vi "Main.vi"() -> ()   [LabVIEW 2026]
doc: "This Continuous Measurement sample project is based on the Queued Message Handler template.\n\nThe Event Handling Loop generates messages based on user interface actions.\n\nThe Message Handling Loop processes messages generated by the Event Handling Loop, or by other messages. There are also Acquisition and Logging message handling loop subVIs, and a chart updating loop."
uses:
  controls/Messaging Payloads/Sensor CoreData.ctl
  controls/Messaging Payloads/Sensor CoreData Cluster.ctl
  controls/UI/Units Enum.ctl
  controls/UI/Signal Enum.ctl
  controls/UI/Settings Cluster.ctl
  controls/UI/Acq Settings.ctl
  Acquisition/Instrument Specifications Configuration.ctl
  Acquisition/Instrument Specifications Cluster Configuration.ctl
  controls/UI/Measurement Role.ctl
  controls/UI/Config Settings.ctl
  Processing/Processing Settings.ctl
  Processing/Test Parameters.ctl
  Processing/Test Parameters Cluster.ctl
  controls/UI/Test Sequence Context.ctl
  controls/UI/Test Sequence Context Cluster.ctl
  controls/UI/Direction.ctl
  controls/UI/Session Identfiers.ctl
  controls/UI/Test Sequence Settings.ctl
  controls/UI/Test Sequence State.ctl
  controls/UI/Test Sequence Enum.ctl
  controls/Controller/Stimulus Settings.ctl
  controls/Controller/Stimulus Outputs.ctl
  controls/Controller/Stimulus Output.ctl
  controls/Controller/Controller Core Data.ctl
  controls/Controller/Stimulus Output Configuration.ctl
  controls/Controller/Stimulus Role.ctl
  controls/UI/UI Data.ctl
  controls/UI/UI State.ctl
  controls/UI/System Config.ctl
  controls/UI/Analog Output.ctl
  Acquisition/Acquisition Payload.ctl
  Acquisition/Acquisition Context.ctl
  support/Architecture/Message Queue/Enqueue Message (Single).vi
  support/Architecture/Message Queue/Enqueue Message (Array).vi
  <vilib>/Utility/error.llb/Error Cluster From Error Code.vi
  <vilib>/ErrorRing/Error Ring.xnode
  support/Architecture/User Event - Stop/User Event - Stop.lvlib
  support/Architecture/Message Queue/Message Queue.lvlib
  Settings/Settings Dialog.vi
  Settings/Settings.lvlib
  Database/Database.lvlib
  Logging/Logging.lvlib
  Processing/Processing_Engine.lvlib
  Acquisition/Acquisition.lvlib
  support/UI Utilities/Login.vi
  Analysis/Analysis Dialog.vi
  Analysis/Analysis.lvlib
panel:
  in  "Stop":bool
  in  "Start":bool
  out "Sensor Information":T1
  in  "Generate Analytics":bool
  in  "Simulation Mode":bool
  in  "Manage Serial Numbers":bool
  out "Data":waveform(dbl)[](graph)
  in  "Settings":bool
  out "Status":string
  in  "Exit":bool
  # "OFF"
  # "Automated Safety Calibration Rig"
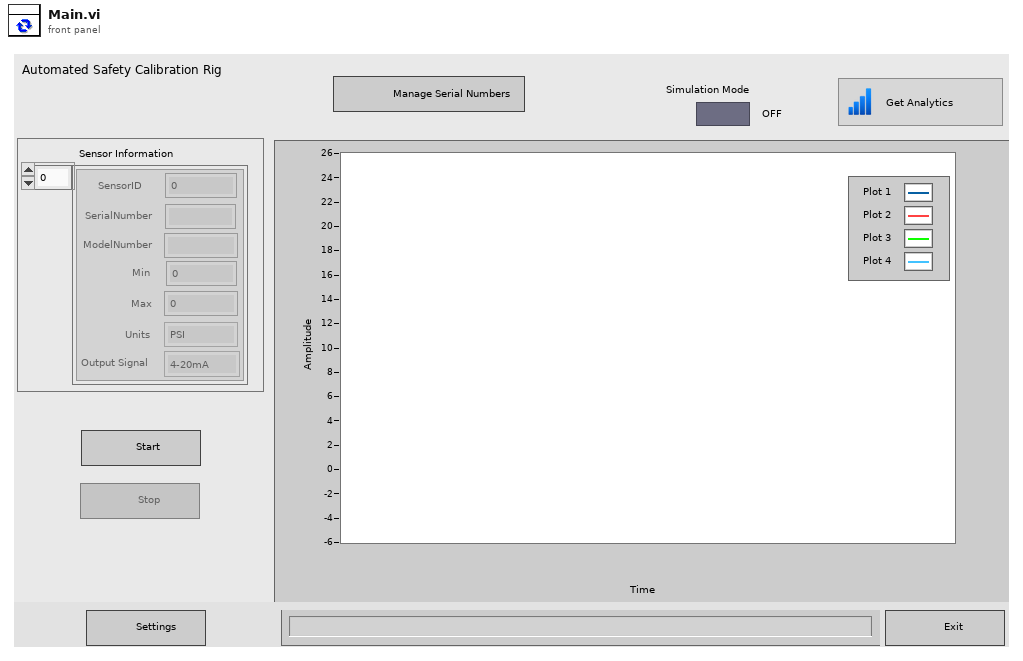
[diagram p1: front panel]
types:
  T1 = typedef "Sensor CoreData.ctl" = T2[]
  T2 = typedef "Settings.lvlib/Sensor CoreData Cluster.ctl" = cluster{"SensorID":i32, "SerialNumber":string, "ModelNumber":string, "Min":dbl, "Max":dbl, "Units":T3, "Output Signal":T4}
  T3 = typedef "Units Enum.ctl" = enum16{"PSI", "Deg C", "kPa", "GPM"}
  T4 = typedef "Signal Enum.ctl" = enum16{"4-20mA", "0-10V", "Thermocouple Type K"}
  T5 = typedef "System Config.ctl" = cluster{"AdminHash":string, "LogFileBasePath ":path, "Config Settings":T6, "AnalogOutput":T7}
  T6 = typedef "Config Settings.ctl" = cluster{"Simulated Sensor Injection":dbl, "Base Device Name":string, "Simulation Mode":string}
  T7 = typedef "Settings.lvlib/Analog Output.ctl" = cluster{"Pressure Controller":string, "Temperature Controller":string}
  T8 = typedef "UI State.ctl" = enum16{"Idle", "Acquiring and Logging", "Waiting for Exit", "Waiting for Exit (Acq Stopped)", "Waiting for Exit (Log Stopped)", "Waiting for Stop", "Waiting for Stop (Acq Stopped)", "Waiting for Stop (Log Stopped)"}
  T9 = typedef "UI Data.ctl" = cluster{"Start Ref":refnum<vi>, "Stop Ref":refnum<vi>, "Settings Ref":refnum<vi>, "Exit Ref":refnum<vi>, "Status Ref":refnum<vi>, "Data Ref":refnum<vi>, "Sim  Refnum":refnum<vi>}
  T10 = typedef "Settings Cluster.ctl" = cluster{"Acq Settings":T11, "Processing Settings":T15, "Session Identifiers":T21, "Test Sequence Settings":T22, "Stimulus Settings":T25}
  T11 = typedef "Acq Settings.ctl" = cluster{"Instrument Specifications":T12, "Config Settings":T6}
  T12 = typedef "Acquisition.lvlib/Instrument Specifications Configuration.ctl" = T13[]
  T13 = typedef "Acquisition.lvlib/Instrument Specifications Cluster Configuration.ctl" = cluster{"Sensor ID":i32, "Target Sample Rate (Hz)":dbl, "Steady-State Duration (s)":i32, "Allowed Tolerance (%) FS":dbl, "Max Settling Timeout (s)":i32, "Physical Channel":string, "Measurement Role":T14}
  T14 = typedef "Settings.lvlib/Measurement Role.ctl" = enum16{"Controller", "Reference", "UUT", "Disable", "All"}
  T15 = typedef "Processing_Engine.lvlib/Processing Settings.ctl" = cluster{"Sensor CoreData":T1, "Test Parameters":T16, "Measurement Roles":T14[], "Test Sequence Context":T18}
  T16 = typedef "Processing_Engine.lvlib/Test Parameters.ctl" = T17[]
  T17 = typedef "Settings.lvlib/Test Parameters Cluster.ctl" = cluster{"Steady-State Duration (s)":i32, "Allowed Tolerance (%) FS":dbl, "Max Settling Timeout (s)":i32}
  T18 = typedef "Settings.lvlib/Test Sequence Context.ctl" = T19[]
  T19 = typedef "Settings.lvlib/Test Sequence Context Cluster.ctl" = cluster{"Direction":T20, "Cycle Number":i32}
  T20 = typedef "Settings.lvlib/Direction.ctl" = enum16{"Acsending", "Descending"}
  T21 = typedef "Session Identfiers.ctl" = cluster{"SerialNumber":string[], "OperatorName":string}
  T22 = typedef "Test Sequence Settings.ctl" = cluster{"Test Sequence State":T23}
  T23 = typedef "Settings.lvlib/Test Sequence State.ctl" = cluster{"Test Sequence Enum":T24, "Point Index":i32, "Current Target":dbl, "Previous Target":dbl, "Simulation?":bool, "Direction":T20, "Transition Active?":bool, "Cycle Number":i32}
  T24 = typedef "Test Sequence Enum.ctl" = enum16{"Idle", "Start Point", "Point Complete", "Test Complete", "Abort Test", "Reset"}
  T25 = typedef "Settings.lvlib/Stimulus Settings.ctl" = cluster{"Stimulus Outputs":T26}
  T26 = typedef "Settings.lvlib/Stimulus Outputs.ctl" = T27[]
  T27 = typedef "Settings.lvlib/Stimulus Output.ctl" = cluster{"Controller Core Data":T28, "Stimulus Output Configuration":T29}
  T28 = typedef "Settings.lvlib/Controller Core Data.ctl" = cluster{"Min":dbl, "Max":dbl, "Units":T3, "Input Signal Type":T4, "Input Signal Min":dbl, "Input Signal Max":dbl}
  T29 = typedef "Settings.lvlib/Stimulus Output Configuration.ctl" = cluster{"DAQmx AO Physical Channel":tag, "Role":T30, "Model Numbers":string, "Serial Numbers":string}
  T30 = typedef "Stimulus Role.ctl" = enum16{"Pressure Controller", "Temperature Controller"}
  T31 = typedef "Message Queue.lvlib/All Message Queues.ctl" = cluster{"UI":refnum<queue>, "Database":refnum<queue>, "Processing":refnum<queue>, "Acquisition":refnum<queue>, "Logging":refnum<queue>, "Analysis":refnum<queue>}
  T32 = enum8{"Enabled", "Disabled", "Disabled and Grayed Out"}
  T33 = typedef "Acquisition.lvlib/Acquisition Payload.ctl" = cluster{"Acq Settings":T11, "Acquisition Context":T34, "Stimulus Settings":T25}
  T34 = typedef "Acquisition.lvlib/Acquisition Context.ctl" = cluster{"Setpoint":dbl, "Previous Setpoint":dbl, "Transition Start Time":dbl, "Transition Active?":bool}
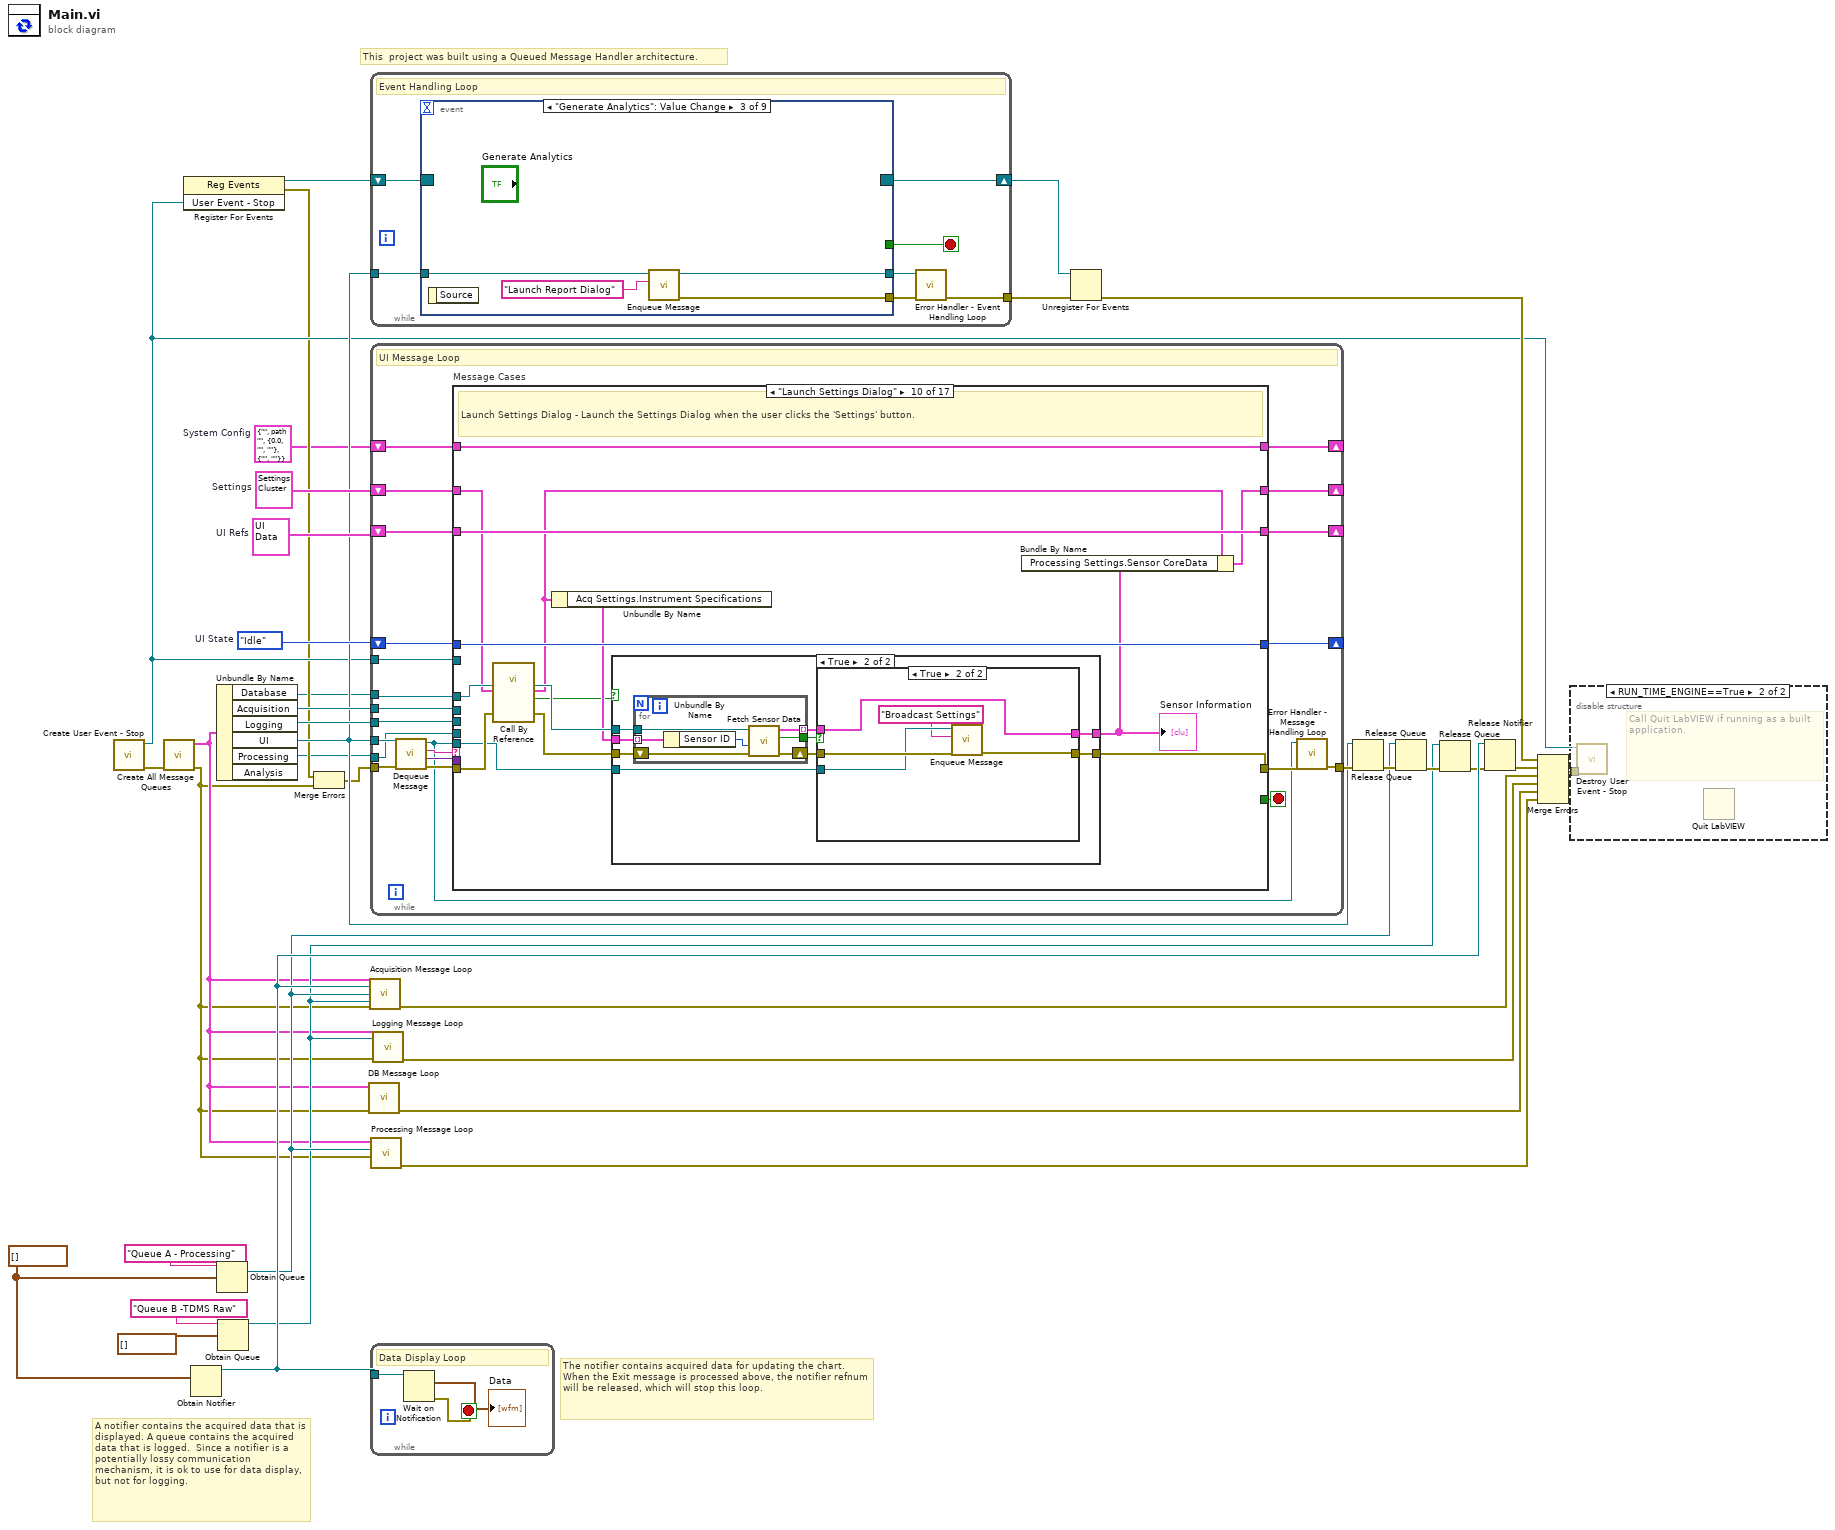
[diagram p0: block diagram]
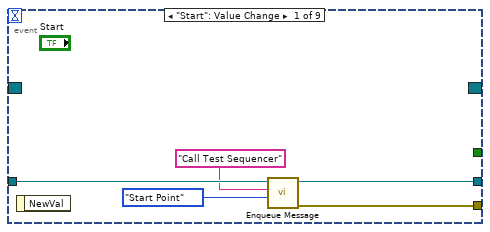
[diagram p3: hidden frame]
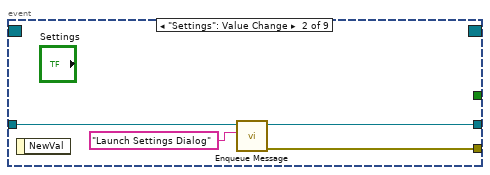
[diagram p4: hidden frame]
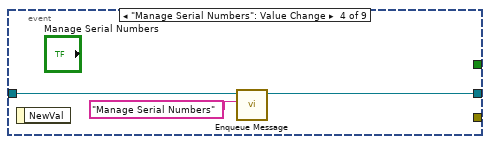
[diagram p5: hidden frame]
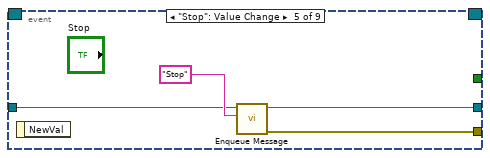
[diagram p6: hidden frame]
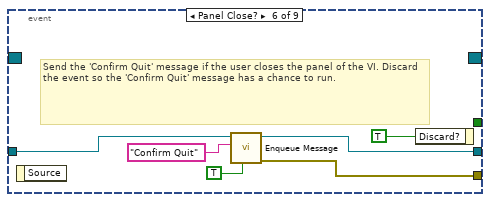
[diagram p7: hidden frame]
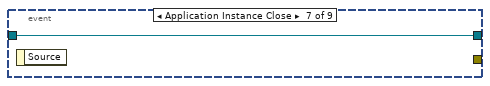
[diagram p8: hidden frame]
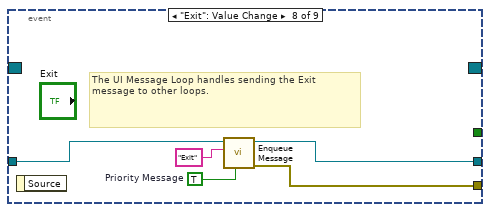
[diagram p9: hidden frame]
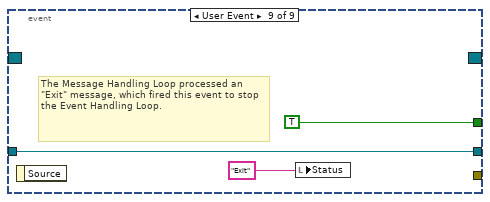
[diagram p10: hidden frame]
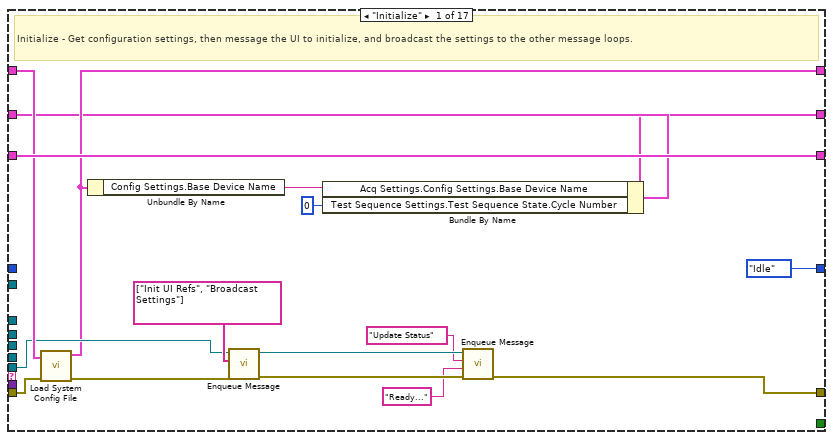
[diagram p11: hidden frame]
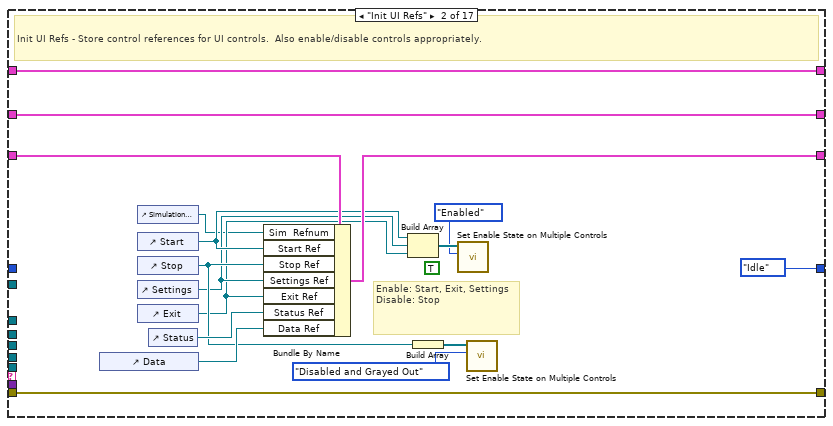
[diagram p12: hidden frame]
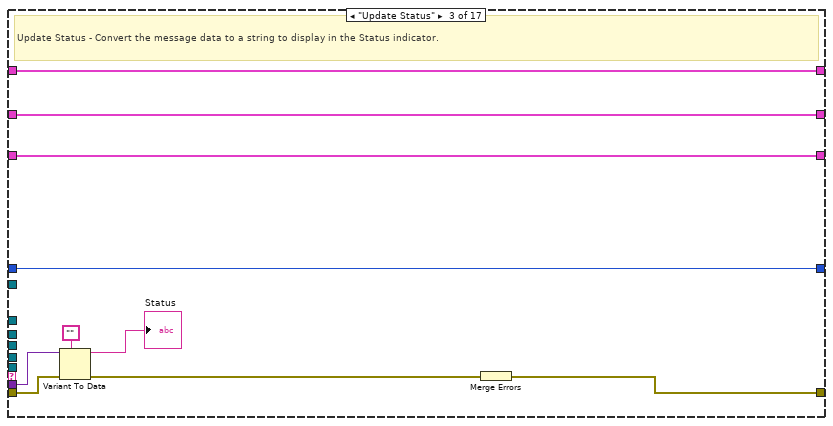
[diagram p13: hidden frame]
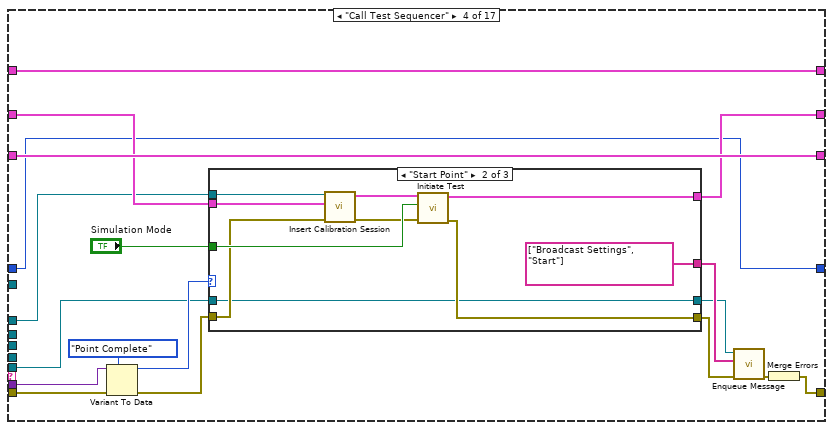
[diagram p14: hidden frame]
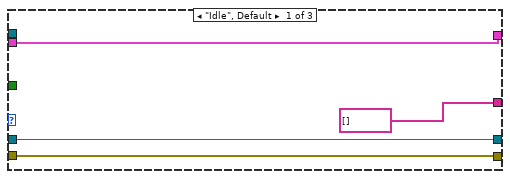
[diagram p15: hidden frame]
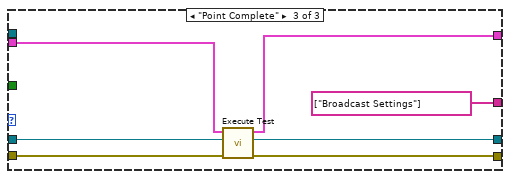
[diagram p16: hidden frame]
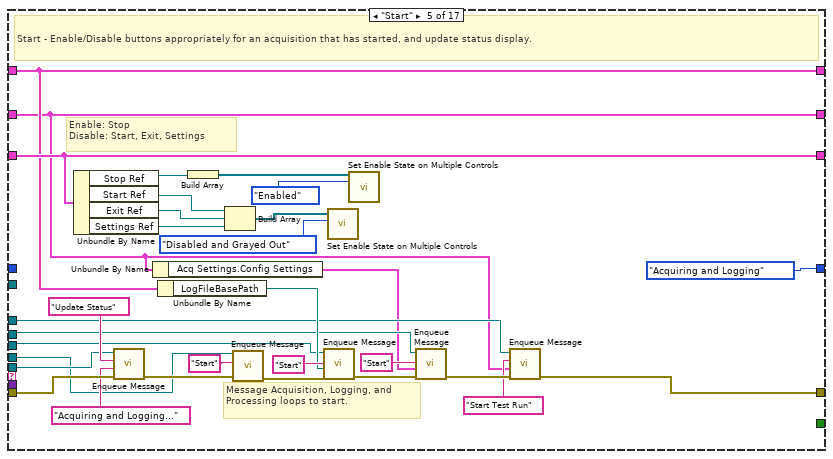
[diagram p17: hidden frame]
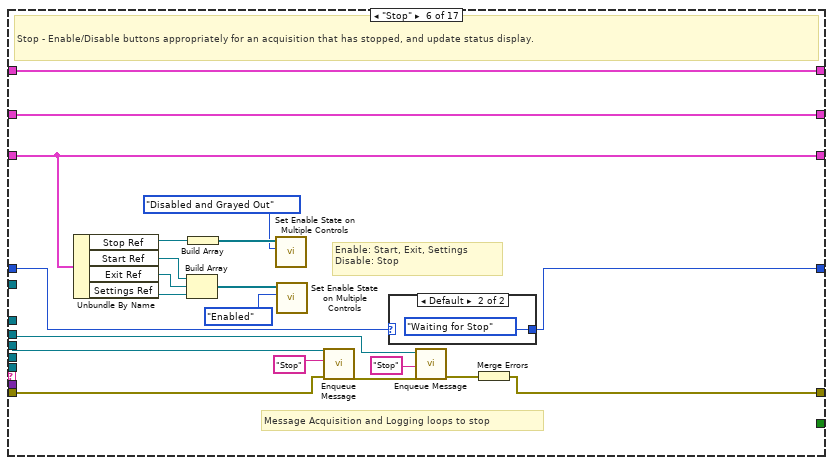
[diagram p18: hidden frame]
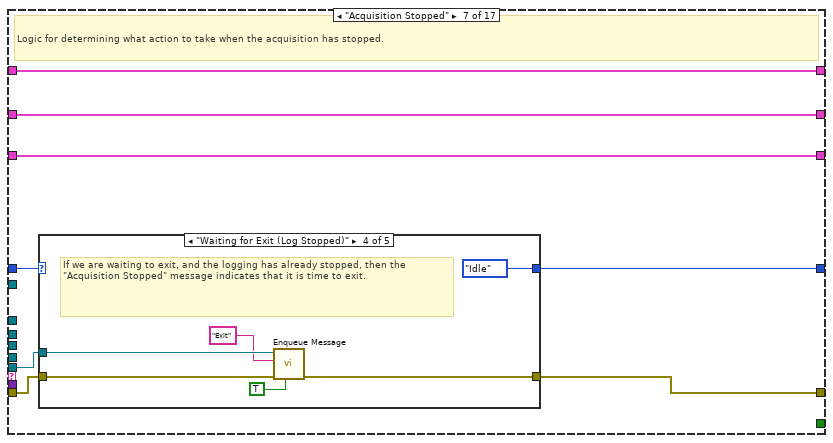
[diagram p20: hidden frame]
diagram:
  w14 = T5 {"AdminHash"="", "LogFileBasePath "=path "", "Config Settings"={"Simulated Sensor Injection"=0.0, "Base Device Name"="", "Simulation Mode"=""}, "AnalogOutput"={"Pressure Controller"="", "Temperature Controller"=""}}  # System Config
  w26 = UI_State."Idle"  # UI State
  w6 = waveform(dbl)[] []
  w29 = T9 {"Start Ref"=refnum, "Stop Ref"=refnum, "Settings Ref"=refnum, "Exit Ref"=refnum, "Status Ref"=refnum, "Data Ref"=refnum, "Sim  Refnum"=refnum}  # UI Refs
  w32 = T10 {"Acq Settings"={"Instrument Specifications"=[], "Config Settings"={"Simulated Sensor Injection"=0.0, "Base Device Name"="", "Simulation Mode"=""}}, "Processing Settings"={"Sensor CoreData"=[], "Test Parameters"=[], "Measurement Roles"=[], "Test Sequence Context"=[]}, "Session Identifiers"={"SerialNumber"=[], "OperatorName"=""}, "Test Sequence Settings"={"Test Sequence State"={"Test Sequence Enum"=enum."Idle", "Point Index"=0, "Current Target"=0.0, "Previous Target"=0.0, "Simulation?"=FALSE, "Direction"=enum."Acsending", "Transition Active?"=FALSE, "Cycle Number"=0}}, "Stimulus Settings"={"Stimulus Outputs"=[]}}  # Settings
  # "This  project was built using a Queued Message Handler architecture."
  # "A notifier contains the acquired data that is displayed. A queue contains the acquired data that is logged.  Since a notifier is a potentially lossy communication mechanism, it is ok to use for data display, but not for logging."
  # "The notifier contains acquired data for updating the chart. When the Exit message is processed above, the notifier refnum will be released, which will stop this loop."
  n1 = call "Create User Event - Stop.vi"() -> ("error out"=w34:errorcluster, "User Event - Stop"=w19:refnum<user-event>)  [unwired: 10 in]
  n2 = call "Create All Message Queues.vi"("error in (no error)"=w34) -> ("error out"=w1:errorcluster, "Message Queues out"=w2:T31)  [unwired: 9 in]
  n3 = register-events(w19) -> (reference out=w20:refnum<event-registration>, error out=w17:errorcluster)  [unwired: 2 in]
  n4 = Obtain Notifier(notification data type=w6) -> (notifier out=w8:refnum<notifier>)  [unwired: 3 in, 2 out]
  n5 = Unbundle By Name(w2) -> ("Database"=w15:refnum<queue>, "Acquisition"=w28:refnum<queue>, "Logging"=w27:refnum<queue>, "UI"=w24:refnum<queue>, "Processing"=w13:refnum<queue>)  [unwired: 1 out]
  n6 = Obtain Queue(name (unnamed)="Queue A - Processing", element data type=w6) -> (queue out=w7:refnum<queue>)  [unwired: 3 in, 2 out]
  n7 = Obtain Queue(name (unnamed)="Queue B -TDMS Raw", element data type=waveform(dbl)[] []) -> (queue out=w3:refnum<queue>)  [unwired: 3 in, 2 out]
  n8 = Merge Errors(w17, w1) -> (w18:errorcluster)
  n9 = call "DB Message Loop.vi"("error in (no error)"=w1, "Message Queues"=w2) -> ("error out"=w16:errorcluster)  [unwired: 9 in]
  n10 = call "Acquisition Message Loop.vi"("Message Queues"=w2, "Data Notifier"=w8, "Queue A - Processing"=w7, "Queue B -TDMS Raw"=w3, "error in (no error)"=w1) -> ("error out"=w35:errorcluster)  [unwired: 10 in]
  n11 = while {
    tunnel: w24 -> [w43]
    tunnel: [w40] -> w36
    shift-right: [w42] -> w30
    shift-left: w20 -> [w44]
    stop <- w41 stop-if-true
    # "Event Handling Loop"
    n12 = event shown="[2] \"Generate Analytics\": Value Change" {
      selector: w44 -> [_ _ _ _ _ _ _ _ _]
      dyn-events: [_ _ _ _ _ _ _ _ _] -> w42
      timeout: _ -> [_ _ _ _ _ _ _ _ _]
      tunnel: [_ _ _ _ _ _ _ _ TRUE ("Discard?")] -> w41
      tunnel: w43 -> [w49 w52 w56 w59 w63 w68 w71 w73 w77]
      tunnel: [w47 w50 w54 _ w62 w66 _ w76 _] -> w39
      tunnel: [w46 w51 w55 w58 w61 w67 w71 w72 w77] -> w38
      event "Start": Value Change {
        n13 = event-data() -> ()  [unwired: 1 in, 1 out]
        n14 = call-poly "Enqueue Message.vi"("Message Data"=Test_Sequence_Enum."Start Point" ("Test Sequence State.Test Sequence Enum"), "Message"="Call Test Sequencer", "Message Queue"=w49) -> ("error out"=w47:errorcluster, "dup Message Queue"=w46:refnum<queue>)  [unwired: 7 in]
      }
      event "Settings": Value Change {
        n15 = event-data() -> ()  [unwired: 1 in, 1 out]
        n16 = call-poly "Enqueue Message.vi"("Message"="Launch Settings Dialog", "Message Queue"=w52) -> ("error out"=w50:errorcluster, "dup Message Queue"=w51:refnum<queue>)  [unwired: 8 in]
      }
      event "Generate Analytics": Value Change {
        n17 = event-data() -> ()  [unwired: 1 in, 1 out]
        n18 = call-poly "Enqueue Message.vi"("Message"="Launch Report Dialog", "Message Queue"=w56) -> ("error out"=w54:errorcluster, "dup Message Queue"=w55:refnum<queue>)  [unwired: 8 in]
      }
      event "Manage Serial Numbers": Value Change {
        n19 = event-data() -> ()  [unwired: 1 in, 1 out]
        n20 = call-poly "Enqueue Message.vi"("Message"="Manage Serial Numbers", "Message Queue"=w59) -> ("dup Message Queue"=w58:refnum<queue>)  [unwired: 8 in, 1 out]
      }
      event "Stop": Value Change {
        n21 = event-data() -> ()  [unwired: 1 in, 1 out]
        n22 = call-poly "Enqueue Message.vi"("Message"="Stop", "Message Queue"=w63) -> ("error out"=w62:errorcluster, "dup Message Queue"=w61:refnum<queue>)  [unwired: 8 in]
      }
      event Panel Close? {
        # "Send the 'Confirm Quit' message if the user closes the panel of the VI. Discard the event so the 'Confirm Quit' message has a chance to run."
        n23 = event-data() -> ()  [unwired: 1 in, 1 out]
        n24 = call-poly "Enqueue Message.vi"("Priority Message? (F)"=TRUE, "Message"="Confirm Quit", "Message Queue"=w68) -> ("error out"=w66:errorcluster, "dup Message Queue"=w67:refnum<queue>)  [unwired: 7 in]
        n25 = event-data("Discard?"=TRUE) -> ()  [unwired: 1 in, 1 out]
      }
      event Application Instance Close {
        n26 = event-data() -> ()  [unwired: 1 in, 1 out]
      }
      event "Exit": Value Change {
        w74 = TRUE  # Priority Message
        # "The UI Message Loop handles sending the Exit message to other loops."
        n27 = event-data() -> ()  [unwired: 1 in, 1 out]
        n28 = call-poly "Enqueue Message.vi"("Priority Message? (F)"=w74, "Message"="Exit", "Message Queue"=w73) -> ("error out"=w76:errorcluster, "dup Message Queue"=w72:refnum<queue>)  [unwired: 7 in]
      }
      event User Event {
        # "The Message Handling Loop processed an \"Exit\" message, which fired this event to stop the Event Handling Loop."
        n29 = event-data() -> ()  [unwired: 1 in, 1 out]
        n30 = local write "Status"("Exit" ("Exit String")) -> ()
      }
    }
    n31 = call "Error Handler - Event Handling Loop.vi"("error in (no error)"=w39, "Message Queue"=w38) -> ("dup error in"=w40:errorcluster)  [unwired: 8 in, 1 out]
  }
  n32 = while {
    tunnel: w24 -> [w95]
    tunnel: w19 -> [w100]
    shift-right: [w94] -> _
    shift-left: w32 -> [w93]
    shift-right: [w91] -> _
    shift-left: w29 -> [w92]
    tunnel: w28 -> [w90]
    tunnel: w27 -> [w89]
    shift-right: [w84] -> _
    shift-left: w26 -> [w85]
    tunnel: w18 -> [w99]
    tunnel: [w88] -> w37
    tunnel: w15 -> [w83]
    shift-right: [w81] -> _
    shift-left: w14 -> [w82]
    tunnel: w13 -> [w80]
    stop <- w101 stop-if-true
    # "UI Message Loop"
    n33 = call "Dequeue Message.vi"("error in (no error)"=w99, "Message Queue"=w95) -> ("error out"=w98:errorcluster, "Message Data"=w96:variant, "Message"=w97:string, "dup Message Queue"=w86:refnum<queue>)  [unwired: 6 in]
    n34 = case "Message Cases" shown="\"Launch Settings Dialog\"" w97 {
      selector: w97 -> [_ _ _ _ _ _ _ _ _ _ _ _ _ _ _ _ w438]
      tunnel: w86 -> [w109 _ _ w148 w192 _ w242 w268 _ w313 _ w368 _ w384 _ _ _]
      tunnel: w98 -> [w111 w135 w144 w163 w215 w236 w243 w269 w302 w326 w359 w369 w371 w383 w415 w435 _]
      tunnel: [w103 w135 w145 w157 w195 w216 w240 w266 w311 w322 w355 w364 w374 w382 w427 w434 w437] -> w87
      tunnel: [_ _ _ _ _ _ _ _ _ _ _ _ _ _ TRUE _ _] -> w101
      tunnel: w96 -> [_ _ w143 w162 _ _ _ _ _ _ _ _ w375 _ w420 _ _]
      tunnel: w100 -> [_ _ _ _ _ _ _ _ _ _ _ _ _ _ w428 _ _]
      tunnel: [w104 w134 w139 w158 w186 w235 w246 w272 w292 w314 w354 w361 w379 w387 w426 w433 w441] -> w94
      tunnel: w93 -> [w105 w134 w139 w156 w186 w235 w246 w272 w301 w320 w354 w361 w379 w387 w426 w433 w441]
      tunnel: w92 -> [w114 w133 w138 w161 w213 w234 w245 w271 w310 w324 w358 w366 w378 w386 w425 w432 w440]
      tunnel: [w114 w130 w138 w161 w213 w234 w245 w271 w310 w324 w358 w366 w378 w386 w425 w432 w440] -> w91
      tunnel: w90 -> [_ _ _ _ w191 w223 _ _ w300 _ _ _ _ _ w417 _ _]
      tunnel: w89 -> [_ _ _ _ w190 w226 _ _ _ _ _ _ _ _ w424 _ _]
      tunnel: w85 -> [_ _ w137 w155 _ w220 w244 w270 w309 w323 w357 w365 w373 w385 _ w431 w439]
      tunnel: [UI_State."Idle" ("UI State") UI_State."Idle" ("UI State") w137 w155 UI_State."Acquiring and Logging" ("UI State") w221 w241 w267 w309 w323 w357 w365 w373 w381 UI_State."Idle" ("UI State") w431 w439] -> w84
      tunnel: w83 -> [_ _ _ w146 w193 _ _ _ _ w321 w353 w360 _ _ w418 _ _]
      tunnel: w82 -> [w110 w122 w136 w160 w202 w219 w239 w265 w308 w319 w356 w363 w370 w380 w414 w430 w436]
      tunnel: [w106 w122 w136 w160 w202 w219 w239 w265 w308 w319 w356 w363 w370 w380 w414 w430 w436] -> w81
      tunnel: w80 -> [_ _ _ _ w189 _ _ _ w306 _ _ _ _ _ w409 _ _]
      frame "Initialize" {
        # "Initialize - Get configuration settings, then message the UI to initialize, and broadcast the settings to the other message loops."
        n35 = call "Load System Config File.vi"("error in (no error)"=w111, "System Config in"=w110) -> ("error out"=w108:errorcluster, "System Config out"=w106:T5)  [unwired: 8 in]
        n36 = Unbundle By Name(w106) -> ("Config Settings.Base Device Name"=w107:string)
        n37 = call-poly "Enqueue Message.vi"("error in (no error)"=w108, "Message Array"=string[] ["Init UI Refs", "Broadcast Settings"], "Message Queue"=w109) -> ("error out"=w118:errorcluster, "dup Message Queue"=w117:refnum<queue>)  [unwired: 7 in]
        n38 = Bundle By Name(cluster=w105, "Acq Settings.Config Settings.Base Device Name"=w107, "Test Sequence Settings.Test Sequence State.Cycle Number"=0) -> (w104:T10)
        n39 = call-poly "Enqueue Message.vi"("error in (no error)"=w118, "Message Data"="Ready..." ("Ready..."), "Message"="Update Status", "Message Queue"=w117) -> ("error out"=w103:errorcluster)  [unwired: 6 in, 1 out]
      }
      frame "Init UI Refs" {
        (unwired) TRUE ("Enable?")
        # "Enable: Start, Exit, Settings\nDisable: Stop"
        # "Init UI Refs - Store control references for UI controls.  Also enable/disable controls appropriately."
        n40 = control-ref of="Data"() -> (w131:refnum<vi>)
        n41 = control-ref of="Simulation Mode"() -> (w121:refnum<vi>)
        n42 = control-ref of="Start"() -> (w126:refnum<vi>)
        n43 = control-ref of="Stop"() -> (w127:refnum<vi>)
        n44 = control-ref of="Settings"() -> (w125:refnum<vi>)
        n45 = control-ref of="Exit"() -> (w124:refnum<vi>)
        n46 = control-ref of="Status"() -> (w132:refnum<vi>)
        n47 = Bundle By Name(cluster=w133, "Sim  Refnum"=w121, "Start Ref"=w126, "Stop Ref"=w127, "Settings Ref"=w125, "Exit Ref"=w124, "Status Ref"=w132, "Data Ref"=w131) -> (w130:T9)
        n48 = Build Array(w126, w125, w124) -> (w129:refnum<vi>[])
        n49 = Build Array(w127) -> (w128:refnum<vi>[])
        n50 = call "Set Enable State on Multiple Controls.vi"("Controls"=w129, "Disabled"=T32."Enabled") -> ()  [unwired: 8 in, 1 out]
        n51 = call "Set Enable State on Multiple Controls.vi"("Controls"=w128, "Disabled"=T32."Disabled and Grayed Out") -> ()  [unwired: 8 in, 1 out]
      }
      frame "Update Status" {
        # "Update Status - Convert the message data to a string to display in the Status indicator."
        n52 = Variant To Data(error in=w144, type="", Variant=w143) -> (data=→"Status":string, error out=w141:errorcluster)
        n53 = Merge Errors(w141) -> (w145:errorcluster)
      }
      frame "Call Test Sequencer" {
        n54 = Variant To Data(error in=w163, type=Test_Sequence_Enum."Point Complete" ("Test Sequence Enum"), Variant=w162) -> (data=w150:T24, error out=w159:errorcluster)
        n55 = case shown="\"Start Point\"" w150 {
          tunnel: w159 -> [w166 w173 w183]
          tunnel: [w166 w177 w182] -> w153
          tunnel: [w167 w176 w181] -> w158
          tunnel: "Simulation Mode" -> [_ w175 _]
          tunnel: w156 -> [w167 w169 w180]
          tunnel: [string[] [] string[] ["Broadcast Settings", "Start"] string[] ["Broadcast Settings"]] -> w152
          tunnel: w148 -> [w164 w171 w179]
          tunnel: [w164 w171 w178] -> w147
          tunnel: w146 -> [_ w168 _]
          frame "Idle", Default {
          }
          frame "Start Point" {
            n56 = call "Insert Calibration Session.vi"("error in (no error)"=w173, "Settings in"=w169, "Database"=w168) -> ("error out"=w172:errorcluster, "Settings out"=w170:T10)  [unwired: 7 in]
            n57 = call "Initiate Test.vi"("error in (no error)"=w172, "Simulation?"=w175, "Settings in"=w170) -> ("error out"=w177:errorcluster, "Settings out"=w176:T10)  [unwired: 7 in]
          }
          frame "Point Complete" {
            n58 = call "Execute Test.vi"("error in (no error)"=w183, "UI in"=w179, "Settings in"=w180) -> ("error out"=w182:errorcluster, "UI out"=w178:refnum<queue>, "Settings out"=w181:T10)  [unwired: 6 in]
          }
        }
        n59 = call-poly "Enqueue Message.vi"("error in (no error)"=w153, "Message Array"=w152, "Message Queue"=w147) -> ("error out"=w154:errorcluster)  [unwired: 7 in, 1 out]
        n60 = Merge Errors(w154) -> (w157:errorcluster)
      }
      frame "Start" {
        # "Message Acquisition, Logging, and \nProcessing loops to start."
        # "Enable: Stop\nDisable: Start, Exit, Settings"
        # "Start - Enable/Disable buttons appropriately for an acquisition that has started, and update status display."
        n61 = Unbundle By Name(w213) -> ("Stop Ref"=w210:refnum<vi>, "Start Ref"=w209:refnum<vi>, "Exit Ref"=w208:refnum<vi>, "Settings Ref"=w207:refnum<vi>)
        n62 = call-poly "Enqueue Message.vi"("error in (no error)"=w215, "Message Data"="Acquiring and Logging..." ("Acquiring and Logging..."), "Message"="Update Status", "Message Queue"=w192) -> ("error out"=w198:errorcluster)  [unwired: 6 in, 1 out]
        n63 = Unbundle By Name(w186) -> ("Acq Settings.Config Settings"=w185:T6)
        n64 = Unbundle By Name(w202) -> ("LogFileBasePath"=w201:path)
        n65 = Build Array(w210) -> (w211:refnum<vi>[])
        n66 = Build Array(w209, w208, w207) -> (w212:refnum<vi>[])
        n67 = call-poly "Enqueue Message.vi"("error in (no error)"=w198, "Message"="Start", "Message Queue"=w189) -> ("error out"=w197:errorcluster)  [unwired: 7 in, 1 out]
        n68 = call-poly "Enqueue Message.vi"("error in (no error)"=w197, "Message Data"=w201, "Message"="Start", "Message Queue"=w190) -> ("error out"=w205:errorcluster)  [unwired: 6 in, 1 out]
        n69 = call "Set Enable State on Multiple Controls.vi"("Controls"=w212, "Disabled"=T32."Disabled and Grayed Out") -> ()  [unwired: 8 in, 1 out]
        n70 = call "Set Enable State on Multiple Controls.vi"("Controls"=w211, "Disabled"=T32."Enabled") -> ()  [unwired: 8 in, 1 out]
        n71 = call-poly "Enqueue Message.vi"("error in (no error)"=w205, "Message Data"=w185, "Message"="Start", "Message Queue"=w191) -> ("error out"=w196:errorcluster)  [unwired: 6 in, 1 out]
        n72 = call-poly "Enqueue Message.vi"("error in (no error)"=w196, "Message Data"=w186, "Message"="Start Test Run", "Message Queue"=w193) -> ("error out"=w195:errorcluster)  [unwired: 6 in, 1 out]
      }
      frame "Stop" {
        # "Message Acquisition and Logging loops to stop"
        # "Enable: Start, Exit, Settings\nDisable: Stop"
        # "Stop - Enable/Disable buttons appropriately for an acquisition that has stopped, and update status display."
        n73 = Unbundle By Name(w234) -> ("Stop Ref"=w231:refnum<vi>, "Start Ref"=w230:refnum<vi>, "Exit Ref"=w229:refnum<vi>, "Settings Ref"=w228:refnum<vi>)
        n74 = Build Array(w230, w229, w228) -> (w233:refnum<vi>[])
        n75 = Build Array(w231) -> (w232:refnum<vi>[])
        n76 = call "Set Enable State on Multiple Controls.vi"("Controls"=w232, "Disabled"=T32."Disabled and Grayed Out") -> ()  [unwired: 8 in, 1 out]
        n77 = call "Set Enable State on Multiple Controls.vi"("Controls"=w233, "Disabled"=T32."Enabled") -> ()  [unwired: 8 in, 1 out]
        n78 = call-poly "Enqueue Message.vi"("error in (no error)"=w236, "Message"="Stop", "Message Queue"=w226) -> ("error out"=w225:errorcluster)  [unwired: 7 in, 1 out]
        n79 = case shown="Default" w220 {
          selector: w220 -> [w237 _]
          tunnel: [w237 UI_State."Waiting for Stop" ("UI State")] -> w221
          frame "Waiting for Exit" {
          }
          frame Default {
          }
        }
        n80 = call-poly "Enqueue Message.vi"("error in (no error)"=w225, "Message"="Stop", "Message Queue"=w223) -> ("error out"=w224:errorcluster)  [unwired: 7 in, 1 out]
        n81 = Merge Errors(w224) -> (w216:errorcluster)
      }
      frame "Acquisition Stopped" {
        # "Logic for determining what action to take when the acquisition has stopped."
        n82 = case shown="\"Waiting for Exit (Log Stopped)\"" w244 {
          selector: w244 -> [w248 _ _ _ _]
          tunnel: w243 -> [w247 w250 w252 w258 w264]
          tunnel: w242 -> [_ _ _ w256 w261]
          tunnel: [w248 UI_State."Waiting for Exit (Acq Stopped)" ("UI State") UI_State."Waiting for Stop (Acq Stopped)" ("UI State") UI_State."Idle" ("UI State") UI_State."Idle" ("UI State")] -> w241
          tunnel: [w247 w250 w252 w257 w262] -> w240
          frame Default {
          }
          frame "Waiting for Exit", "Waiting for Exit (Acq Stopped)" {
          }
          frame "Waiting for Stop", "Waiting for Stop (Acq Stopped)" {
          }
          frame "Waiting for Exit (Log Stopped)" {
            # "If we are waiting to exit, and the logging has already stopped, then the \"Acquisition Stopped\" message indicates that it is time to exit."
            n83 = call-poly "Enqueue Message.vi"("Priority Message? (F)"=TRUE, "error in (no error)"=w258, "Message"="Exit", "Message Queue"=w256) -> ("error out"=w257:errorcluster)  [unwired: 6 in, 1 out]
          }
          frame "Waiting for Stop (Log Stopped)" {
            # "If we are waiting to stop, and the logging has already stopped, then the \"Acquisition Stopped\" message indicates that it is time to stop."
            n84 = call-poly "Enqueue Message.vi"("error in (no error)"=w264, "Message Data"="Ready..." ("Ready..."), "Message"="Update Status", "Message Queue"=w261) -> ("error out"=w262:errorcluster)  [unwired: 6 in, 1 out]
          }
        }
      }
      frame "Logging Stopped" {
        # "Logic for determining what action to take when the logging has stopped."
        n85 = case shown="\"Waiting for Exit (Acq Stopped)\"" w270 {
          selector: w270 -> [w274 _ _ _ _]
          tunnel: w269 -> [w273 w276 w278 w284 w287]
          tunnel: w268 -> [_ _ _ w282 w286]
          tunnel: [w274 UI_State."Waiting for Exit (Log Stopped)" ("UI State") UI_State."Waiting for Stop (Log Stopped)" ("UI State") UI_State."Idle" ("UI State") UI_State."Idle" ("UI State")] -> w267
          tunnel: [w273 w276 w278 w283 w285] -> w266
          frame Default {
          }
          frame "Waiting for Exit", "Waiting for Exit (Log Stopped)" {
          }
          frame "Waiting for Stop", "Waiting for Stop (Log Stopped)" {
          }
          frame "Waiting for Exit (Acq Stopped)" {
            # "If we are waiting to exit, and the acquisition has already stopped, then the \"Logging Stopped\" message indicates that it is time to exit."
            n86 = call-poly "Enqueue Message.vi"("Priority Message? (F)"=TRUE, "error in (no error)"=w284, "Message"="Exit", "Message Queue"=w282) -> ("error out"=w283:errorcluster)  [unwired: 6 in, 1 out]
          }
          frame "Waiting for Stop (Acq Stopped)" {
            # "If we are waiting to stop, and the acquisition has already stopped, then the \"Logging Stopped\" message indicates that it is time to stop."
            n87 = call-poly "Enqueue Message.vi"("error in (no error)"=w287, "Message Data"="Ready..." ("Ready..."), "Message"="Update Status", "Message Queue"=w286) -> ("error out"=w285:errorcluster)  [unwired: 6 in, 1 out]
          }
        }
      }
      frame "Broadcast settings" {
        w299 = T33 {"Acq Settings"={"Instrument Specifications"=[], "Config Settings"={"Simulated Sensor Injection"=0.0, "Base Device Name"="", "Simulation Mode"=""}}, "Acquisition Context"={"Setpoint"=0.0, "Previous Setpoint"=0.0, "Transition Start Time"=0.0, "Transition Active?"=FALSE}, "Stimulus Settings"={"Stimulus Outputs"=[]}}  # Acquisition Payload
        # "Broadcast settings - Send the 'Update Settings' message to the Acquisition message loop."
        n88 = call "Create Processing Payload.vi"("error in (no error)"=w302, "Settings in"=w301) -> ("error out"=w296:errorcluster, "Processing Settings"=w294:T15, "Settings out"=w292:T10)  [unwired: 7 in]
        n89 = Unbundle By Name(w292) -> ("Acq Settings"=w298:T11, "Test Sequence Settings.Test Sequence State.Current Target"=w297:dbl, "Test Sequence Settings.Test Sequence State.Previous Target"=w295:dbl, "Test Sequence Settings.Test Sequence State.Transition Active?"=w291:bool)
        n90 = Bundle By Name(cluster=w299, "Acq Settings"=w298, "Acquisition Context.Setpoint"=w297, "Acquisition Context.Previous Setpoint"=w295, "Acquisition Context.Transition Active?"=w291) -> (w293:T33)
        n91 = call-poly "Enqueue Message.vi"("error in (no error)"=w296, "Message Data"=w294, "Message"="Update Settings", "Message Queue"=w306) -> ("error out"=w305:errorcluster)  [unwired: 6 in, 1 out]
        n92 = call-poly "Enqueue Message.vi"("error in (no error)"=w305, "Message Data"=w293, "Message"="Update Settings", "Message Queue"=w300) -> ("error out"=w304:errorcluster)  [unwired: 6 in, 1 out]
        n93 = Merge Errors(w304) -> (w311:errorcluster)
      }
      frame "Launch Settings Dialog" {
        # "Launch Settings Dialog - Launch the Settings Dialog when the user clicks the 'Settings' button."
        n94 = call-by-ref "?"("Settings in"=w320, "Database in"=w321, "error in (no error)"=w326) -> ("Database out"=w318:refnum<queue>, "Settings out"=w315:T10, "UI Refresh Needed?"=w316:bool, "error out"=w325:errorcluster)  [unwired: 9 in, 4 out]
        n95 = Unbundle By Name(w315) -> ("Acq Settings.Instrument Specifications"=w317:T12)
        n96 = case shown="True" w316 {
          tunnel: w325 -> [w328 w337]
          tunnel: [w328 w333] -> w322
          tunnel: w318 -> [_ w336]
          tunnel: [w327 w332] -> w312
          tunnel: w317 -> [_ w329]
          tunnel: w313 -> [_ w330]
          frame False {
            w327 = T1 []  # Sensor CoreData
          }
          frame True {
            n97 = for {
              tunnel: w336 -> [w343]
              tunnel: [w342] -> w335
              tunnel: [w338] -> w331 mode=indexing
              tunnel: w329 -> [w340] mode=indexing
              shift-right: [w341] -> w334
              shift-left: w337 -> [w344]
              n98 = Unbundle By Name(w340) -> ("Sensor ID"=w339:i32)
              n99 = call "Fetch Sensor Data.vi"("error in (no error)"=w344, "SensorID"=w339, "Database"=w343) -> ("error out"=w341:errorcluster, "Data Valid?"=w342:bool, "Sensor CoreData Cluster"=w338:T2)  [unwired: 6 in]
            }
            n100 = case shown="True" w335 {
              tunnel: w334 -> [w346 w352]
              tunnel: [w346 w351] -> w333
              tunnel: [w345 w350] -> w332
              tunnel: w331 -> [_ w350]
              tunnel: w330 -> [_ w349]
              frame False {
                w345 = T1 []  # Sensor CoreData
                n101 = One Button Dialog(message="Error: The Database failed to return the\nSensor Profile. Please verify the Serial\nNumber or check the database connection.") -> ()  [unwired: 1 in, 1 out]
              }
              frame True {
                n102 = call-poly "Enqueue Message.vi"("error in (no error)"=w352, "Message"="Broadcast Settings", "Message Queue"=w349) -> ("error out"=w351:errorcluster)  [unwired: 7 in, 1 out]
              }
            }
          }
        }
        "Sensor Information" <- w312
        n103 = Bundle By Name(cluster=w315, "Processing Settings.Sensor CoreData"=w312) -> (w314:T10)
      }
      frame "Launch Report Dialog" {
        # "Launch Settings Dialog - Launch the Settings Dialog when the user clicks the 'Settings' button."
        n104 = call-by-ref "?"("error in (no error)"=w359, "Database in"=w353) -> ("error IO"=w355:errorcluster)  [unwired: 10 in, 3 out]
      }
      frame "Manage Serial Numbers" {
        # "Manage Serial Numbers Dialog - Launch the Manage Serial Numbers Dialog when the user clicks the 'Manage Serial Numbers' button."
        n105 = call-by-ref "?"("Database"=w360, "error in (no error)"=w369, "System Config"=w363) -> ("error out"=w367:errorcluster)  [unwired: 9 in, 3 out]
        n106 = call-poly "Enqueue Message.vi"("error in (no error)"=w367, "Message"="Broadcast Settings", "Message Queue"=w368) -> ("error out"=w364:errorcluster)  [unwired: 7 in, 1 out]
      }
      frame "Error" {
        # "Error - Display an error dialog. This message is sent by the \"Error Handler\" VIs at the end of other loops in this application."
        n107 = Variant To Data(error in=w371, type=errorcluster {"status"=FALSE, "code"=0, "source"=""} ("error constant"), Variant=w375) -> (data=w372:errorcluster, error out=w376:errorcluster)
        n108 = call <vilib>:"Simple Error Handler.vi"("error in (no error)"=w372) -> ()  [unwired: 4 in, 5 out]
        n109 = Merge Errors(w376) -> (w374:errorcluster)
      }
      frame "Confirm Quit" {
        # "Confirm Quit - Message that can confirm whether or not the user wants to exit the application."
        n110 = case shown="\"Acquiring and Logging\"" w385 {
          tunnel: w384 -> [w393 w397]
          tunnel: w383 -> [w392 w396]
          tunnel: [w391 w395] -> w382
          tunnel: [UI_State."Idle" ("UI State") w394] -> w381
          frame Default {
            # "If 'Confirm Quit' comes in while the system is idle, there is no need for a confirmation message."
            n111 = call-poly "Enqueue Message.vi"("Priority Message? (F)"=TRUE, "error in (no error)"=w392, "Message"="Exit", "Message Queue"=w393) -> ("error out"=w391:errorcluster)  [unwired: 6 in, 1 out]
          }
          frame "Acquiring and Logging" {
            n112 = Two Button Dialog(message="Are you sure you want to quit while the acquisition is running?" ("Confirm Quit Message"), 1:"No" ("No"), 2:"Yes" ("Yes")) -> (T button?=w398:bool)
            n113 = case shown="True" w398 {
              tunnel: w397 -> [_ w407]
              tunnel: w396 -> [w403 w408]
              tunnel: [w403 w406] -> w395
              tunnel: [UI_State."Acquiring and Logging" ("UI State") UI_State."Waiting for Exit" ("UI State")] -> w394
              frame False {
                # "User did not want to quit."
              }
              frame True {
                n114 = call-poly "Enqueue Message.vi"("error in (no error)"=w408, "Message"="Stop", "Message Queue"=w407) -> ("error out"=w406:errorcluster)  [unwired: 7 in, 1 out]
              }
            }
          }
        }
      }
      frame "Exit" {
        w411 = TRUE ("Priority Message? (F)")
        w410 = "Exit" ("Message")
        # "Popup an error dialog if 'Exit' was called as a result of an error."
        # "Stop the VI"
        # "Exit - Send Exit messages to the Acquisition and Logging loops, and fire the user event to stop the Event Handling Loop."
        n115 = call-poly "Enqueue Message.vi"("Priority Message? (F)"=w411, "error in (no error)"=w415, "Message"=w410, "Message Queue"=w418) -> ("error out"=w416:errorcluster)  [unwired: 6 in, 1 out]
        n116 = Variant To Data(type=errorcluster {"status"=FALSE, "code"=0, "source"=""} ("error constant"), Variant=w420) -> (data=w419:errorcluster)  [unwired: 1 in, 1 out]
        n117 = call <vilib>:"Simple Error Handler.vi"("error in (no error)"=w419) -> ()  [unwired: 4 in, 5 out]
        n118 = call-poly "Enqueue Message.vi"("Priority Message? (F)"=w411, "error in (no error)"=w416, "Message"=w410, "Message Queue"=w417) -> ("error out"=w422:errorcluster)  [unwired: 6 in, 1 out]
        n119 = call-poly "Enqueue Message.vi"("Priority Message? (F)"=w411, "error in (no error)"=w422, "Message"=w410, "Message Queue"=w424) -> ("error out"=w413:errorcluster)  [unwired: 6 in, 1 out]
        n120 = call-poly "Enqueue Message.vi"("Priority Message? (F)"=w411, "error in (no error)"=w413, "Message"=w410, "Message Queue"=w409) -> ("error out"=w412:errorcluster)  [unwired: 6 in, 1 out]
        n121 = call "Fire User Event - Stop.vi"("error in (no error)"=w412, "User Event - Stop"=w428) -> ("error out"=w427:errorcluster)  [unwired: 9 in]
      }
      frame "---Copy This Frame---" {
        # "Duplicate this frame when creating new messages.  Change this comment in the duplicated frame to describe this message."
        n122 = Merge Errors(w435) -> (w434:errorcluster)
      }
      frame Default {
        # "'Default' case only runs if there is a message that isn't defined in any of the other cases.  Output a programming error."
        n123 = xnode "Error Ring"("parameter 0"=w438) -> ("error out"=w437:errorcluster)
      }
    }
    n124 = call "Error Handler - Message Handling Loop.vi"("error in (no error)"=w87, "Message Queue"=w86) -> ("dup error in"=w88:errorcluster)  [unwired: 8 in, 1 out]
  }
  n125 = call "Processing Message Loop.vi"("error in (no error)"=w1, "Queue A - Processing"=w7, "Message Queues"=w2) -> ("error out"=w12:errorcluster)  [unwired: 8 in]
  n126 = while "Data Display Loop" {
    tunnel: w8 -> [w451]
    stop <- w449 stop-if-true
    # "Data Display Loop"
    n127 = Wait on Notification(notifier=w451) -> (notification=→"Data":waveform(dbl)[], error out=w449:errorcluster)  [unwired: 3 in, 2 out]
  }
  n128 = call "Logging Message Loop.vi"("error in (no error)"=w1, "Queue B -TDMS Raw"=w3, "Message Queues"=w2) -> ("error out"=w33:errorcluster)  [unwired: 8 in]
  n129 = Unregister For Events(event registration refnum=w30, error in=w36) -> (error out=w31:errorcluster)
  n130 = Release Queue(queue=w24, error in (no error)=w37) -> (error out=w22:errorcluster)  [unwired: 1 in, 2 out]
  n131 = Release Queue(queue=w7, error in (no error)=w22) -> (error out=w5:errorcluster)  [unwired: 1 in, 2 out]
  n132 = Release Queue(queue=w3, error in (no error)=w5) -> (error out=w4:errorcluster)  [unwired: 1 in, 2 out]
  n133 = Release Notifier(notifier=w8, error in (no error)=w4) -> (error out=w21:errorcluster)  [unwired: 1 in, 2 out]
  n134 = Merge Errors(w31, w21, w35, w33, w16, w12) -> (w25:errorcluster)
  n135 = call "Destroy User Event - Stop.vi"("error in (no error)"=w25, "User Event - Stop"=w19) -> ("error out"=w23:errorcluster)  [unwired: 9 in]
  n136 = disable-structure shown="RUN_TIME_ENGINE==True" {
    disable-tunnel: w23 -> [_ _]
    frame condition #0 (active) {
    }
    frame condition #1 {
      # "Call Quit LabVIEW if running as a built application."
      n137 = Quit LabVIEW() -> ()  [unwired: 1 in]
    }
  }
